vi "create transfer specification.vi"(8 "error in":errorcluster, 9 "mapping specification":T3[](array[typedef]), 10 "data dictionary source in":refnum<class "data bus dictionary.lvclass">, 11 "data dictionary sink in":refnum<class "data bus dictionary.lvclass">) -> (0 "error out":errorcluster, 1 "transfer specification":T1[](array[typedef]), 2 "data dictionary source out":refnum<class "data bus dictionary.lvclass">, 3 "data dictionary sink out":refnum<class "data bus dictionary.lvclass">)   [LabVIEW 2013, in "data bus dictionary.lvclass"]
doc: "Uses two data dictionaries and a set of tag names and types to create a transfer specification. This transfer specification can be used to move data from one table to another table. These tables do not need to share the same tags."
uses:
  data bus dictionary.lvclass
  table/mapping specification.ctl
  tag/Data Type.ctl
  table/mapping.ctl
  table/transfer specification.ctl
  tag/data bus tag description.lvclass
  table/data bus values.lvlib
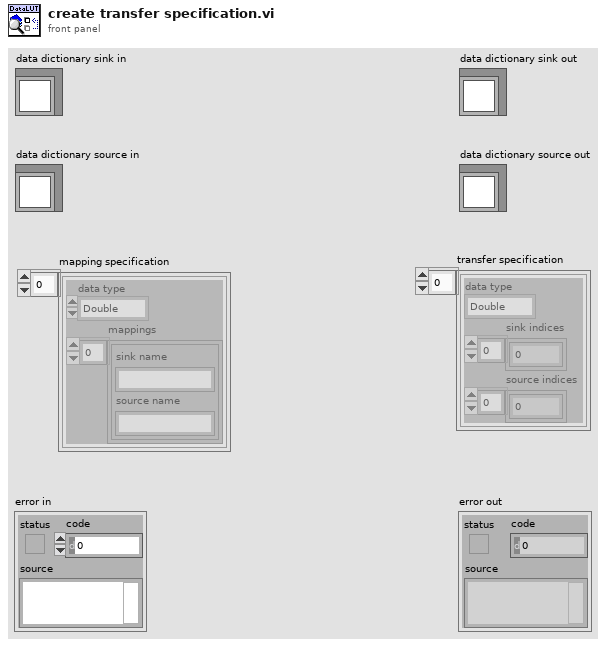
[diagram p1: front panel]
types:
  T1 = typedef "data bus values.lvlib/transfer specification.ctl" = cluster{"data type":T2, "sink indices":i32[], "source indices":i32[]}
  T2 = typedef "data bus tag description.lvclass/Data Type.ctl" = enum16{"Double", "I64", "Boolean", "Array of Double", "Array of I64", "Variant"}
  T3 = typedef "data bus values.lvlib/mapping specification.ctl" = cluster{"data type":T2, "mappings":T4[]}
  T4 = typedef "data bus values.lvlib/mapping.ctl" = cluster{"sink name":string, "source name":string}
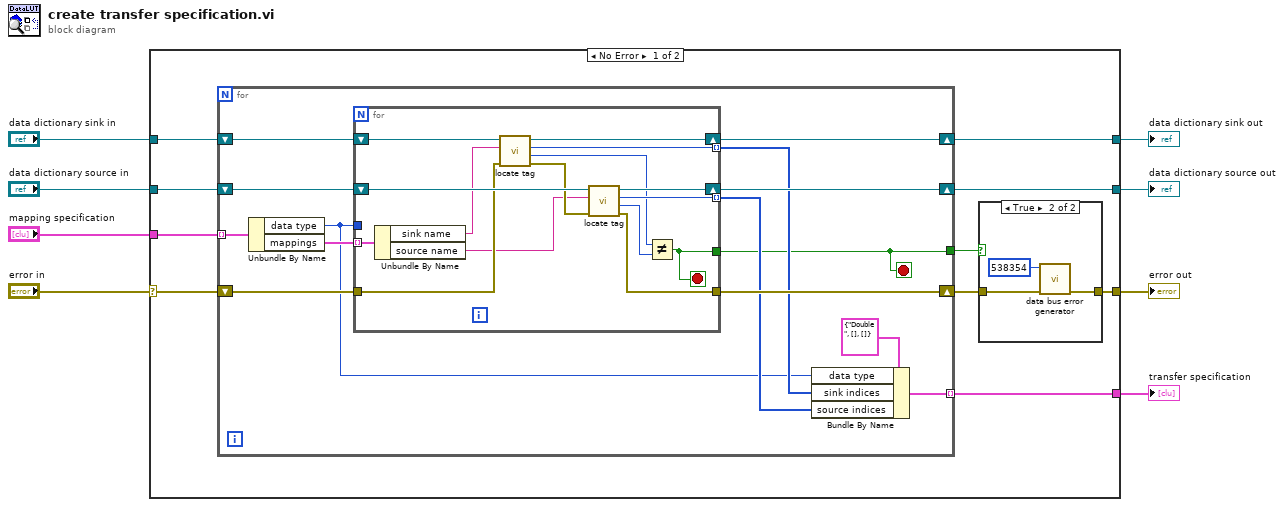
[diagram p0: block diagram]
diagram:
  n1 = case shown="No Error" "error in" {
    selector: "error in" -> [w13 w54]
    tunnel: [w10 w54] -> w7
    tunnel: [w17 w53] -> w5
    tunnel: "data dictionary sink in" -> [w18 w53]
    tunnel: "data dictionary source in" -> [w16 w52]
    tunnel: "mapping specification" -> [w14 _]
    tunnel: [w15 w52] -> w2
    tunnel: [w12 _] -> w1
    frame No Error {
      n2 = for {
        tunnel: w14 -> [w36] mode=indexing
        shift-right: [w30] -> w9
        shift-left: w13 -> [w31]
        tunnel: [w24] -> w12 mode=indexing
        shift-right: [w34] -> w17
        shift-left: w18 -> [w35]
        shift-right: [w32] -> w15
        shift-left: w16 -> [w33]
        tunnel: [w23] -> w11
        stop <- w23 stop-if-true
        n3 = Unbundle By Name(w36) -> ("data type"=w25:T2, "mappings"=w29:T4[])
        n4 = for {
          tunnel: w31 -> [w47]
          tunnel: [w45] -> w30
          tunnel: w29 -> [w44] mode=indexing
          tunnel: w25 -> [_]
          tunnel: [w41] -> w27 mode=indexing
          tunnel: [w40] -> w26 mode=indexing
          shift-right: [w50] -> w34
          shift-left: w35 -> [w51]
          shift-right: [w48] -> w32
          shift-left: w33 -> [w49]
          tunnel: [w37] -> w23
          stop <- w37 stop-if-true
          n5 = Unbundle By Name(w44) -> ("sink name"=w43:string, "source name"=w42:string)
          n6 = call "locate tag.vi"("error in"=w47, "name"=w43, "data dictionary in"=w51) -> ("error out"=w46:errorcluster, "data type"=w39:T2, "index"=w41:i32, "data dictionary out"=w50:refnum<class "data bus dictionary.lvclass">)  [unwired: 5 in]
          n7 = call "locate tag.vi"("error in"=w46, "name"=w42, "data dictionary in"=w49) -> ("error out"=w45:errorcluster, "data type"=w38:T2, "index"=w40:i32, "data dictionary out"=w48:refnum<class "data bus dictionary.lvclass">)  [unwired: 5 in]
          n8 = Not Equal?(x=w39, y=w38) -> (x != y?=w37:bool)
        }
        n9 = Bundle By Name(cluster=T1 {"data type"=enum."Double", "sink indices"=[], "source indices"=[]} ("merge specification"), "data type"=w25, "sink indices"=w27, "source indices"=w26) -> (w24:T1)
      }
      n10 = case shown="True" w11 {
        tunnel: [w19 w21] -> w10
        tunnel: w9 -> [w19 w22]
        frame False {
        }
        frame True {
          n11 = call "data bus error generator.vi"("error in"=w22, "error code (0)"=538354) -> ("error out"=w21:errorcluster)  [unwired: 7 in]
        }
      }
    }
    frame Error {
    }
  }
  "error out" <- w7
  "data dictionary sink out" <- w5
  "data dictionary source out" <- w2
  "transfer specification" <- w1
